vi "queryPanels (SubVI).vi"(4 "ThreatSize_0":refnum<vi>, 6 "Requestors_0":refnum<vi>, 7 "append":bool, 8 "error in":errorcluster, 9 "srchParams":T2={"maxPanels"=1001, "lkupPanelStartDate"=timestamp(0 s since 1904-01-01), "lkupPanelEndDate"=timestamp(0 s since 1904-01-01)} caption="Search Params" {"lkupPanelEndDate" format="%<%x>T"; "lkupPanelStartDate" format="%<%x>T"; "maxPanels" min=1 max=10000 step=100}, 10 "recoSet_IN":string[][](array[string]), 11 "criteria":T1) -> (0 "error out":errorcluster, 2 "recoSet_OUT":string[][](array[string]), 3 "actualNumPanels":i32)   [LabVIEW 2015]
panel:
  out "queryStr":string
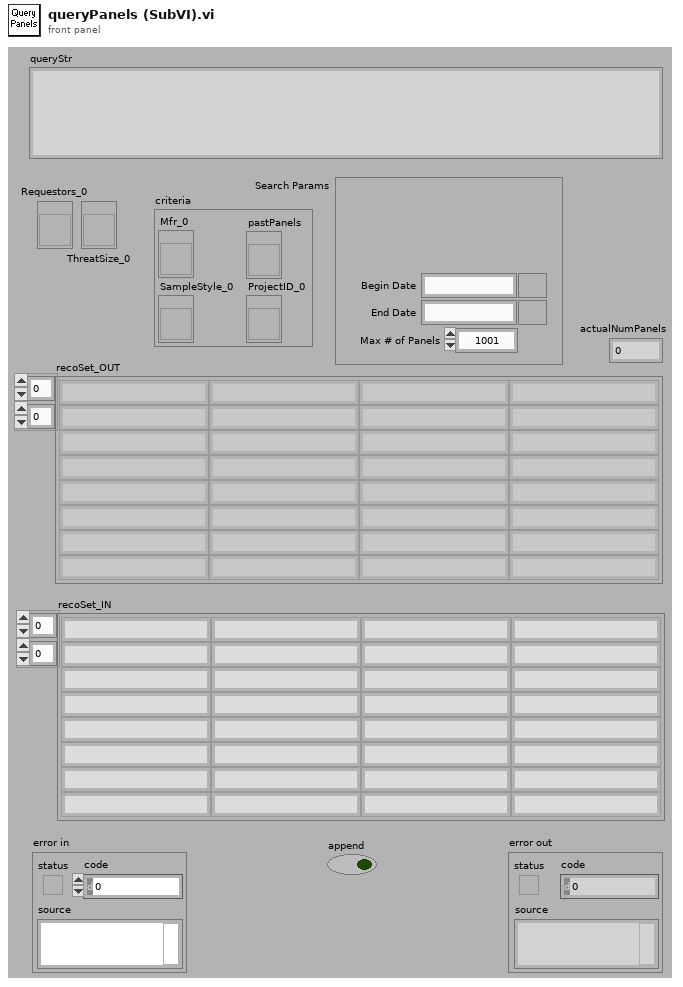
[diagram p1: front panel]
types:
  T1 = cluster{"Mfr_0":refnum<vi>, "SampleStyle_0":refnum<vi>, "pastPanels":refnum<vi>, "ProjectID_0":refnum<vi>}
  T2 = cluster{"maxPanels":u16, "lkupPanelStartDate":timestamp, "lkupPanelEndDate":timestamp}
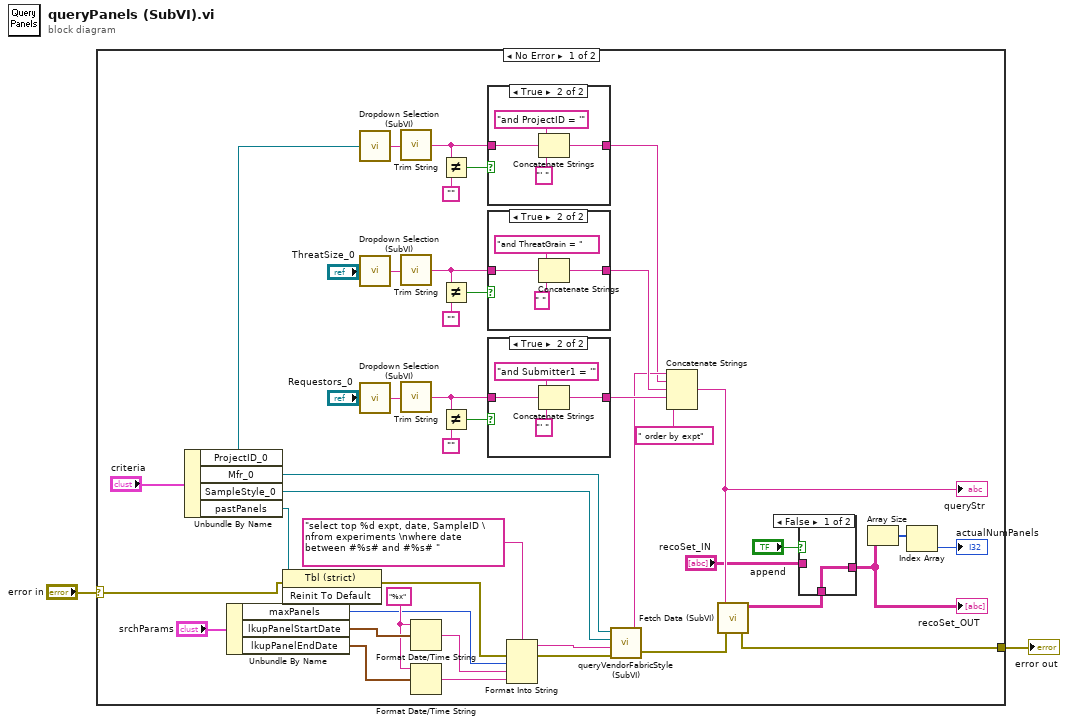
[diagram p0: block diagram]
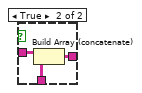
[diagram p2: hidden frame]
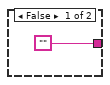
[diagram p3: hidden frame]
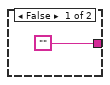
[diagram p4: hidden frame]
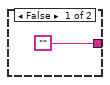
[diagram p5: hidden frame]
diagram:
  n1 = case shown="No Error" "error in" {
    selector: "error in" -> [w31 w67]
    tunnel: [w42 w67] -> w2
    frame No Error {
      w44 = "%x" ("time format string (%c)")
      n2 = Unbundle By Name("criteria") -> ("ProjectID_0"=w3:refnum<vi>, "Mfr_0"=w6:refnum<vi>, "SampleStyle_0"=w5:refnum<vi>, "pastPanels"=w4:refnum<vi>)
      n3 = Unbundle By Name("srchParams") -> ("maxPanels"=w38:u16, "lkupPanelStartDate"=w46:timestamp, "lkupPanelEndDate"=w47:timestamp)
      n4 = invoke class="Tbl (strict)" method="Reinit To Default"(reference=w4, error in=w31) -> (error out=w37:errorcluster)  [unwired: 1 in, 2 out]
      n5 = call "Dropdown Selection (SubVI).vi"("reference"=w3) -> ("element"=w17:string)
      n6 = call "Dropdown Selection (SubVI).vi"("reference"="ThreatSize_0") -> ("element"=w20:string)
      n7 = call "Dropdown Selection (SubVI).vi"("reference"="Requestors_0") -> ("element"=w29:string)
      n8 = call "Trim String.vi"("inStr"=w17) -> ("outStr"=w15:string)
      n9 = call "Trim String.vi"("inStr"=w20) -> ("outStr"=w22:string)
      n10 = call "Trim String.vi"("inStr"=w29) -> ("outStr"=w26:string)
      n11 = Format Date/Time String(time format string (%c)=w44, seconds (now)=w46) -> (date/time string=w39:string)  [unwired: 1 out]
      n12 = Format Date/Time String(time format string (%c)=w44, seconds (now)=w47) -> (date/time string=w40:string)  [unwired: 1 out]
      n13 = Not Equal?(x=w15, y="") -> (x != y?=w14:bool)
      n14 = Not Equal?(x=w22, y="") -> (x != y?=w23:bool)
      n15 = Not Equal?(x=w26, y="") -> (x != y?=w24:bool)
      n16 = case shown="True" w14 {
        tunnel: w15 -> [_ w54]
        tunnel: ["" w53] -> w12
        frame False {
        }
        frame True {
          n17 = Concatenate Strings("and ProjectID = '" ("Format String"), w54, "' " ("Format String")) -> (w53:string)
        }
      }
      n18 = case shown="True" w23 {
        tunnel: w22 -> [_ w59]
        tunnel: ["" w58] -> w18
        frame False {
        }
        frame True {
          n19 = Concatenate Strings("and ThreatGrain = " ("Format String"), w59, " " ("Format String")) -> (w58:string)
        }
      }
      n20 = case shown="True" w24 {
        tunnel: w26 -> [_ w64]
        tunnel: ["" w63] -> w25
        frame False {
        }
        frame True {
          n21 = Concatenate Strings("and Submitter1 = '" ("Format String"), w64, "' " ("Format String")) -> (w63:string)
        }
      }
      n22 = Format Into String(format string="select top %d expt, date, SampleID \nfrom experiments \nwhere date between #%s# and #%s# " ("Format String"), error in=w37, w38, w39, w40) -> (resulting string=w32:string, error out=w33:errorcluster)  [unwired: 1 in]
      n23 = call "queryVendorFabricStyle (SubVI).vi"("errorIn"=w33, "queryInStr"=w32, "SampleStyle_0"=w5, "Mfr_0"=w6) -> ("errorOut"=w34:errorcluster, "queryOutStr"=w13:string)
      n24 = Concatenate Strings(w13, w12, w18, w25, " order by expt" ("Format String")) -> (w35:string)
      "queryStr" <- w35
      n25 = call "Fetch Data (SubVI).vi"("error IN"=w34, "query string"=w35) -> ("error OUT"=w42:errorcluster, "recordset data"=w11:string[][])  [unwired: 4 out]
      n26 = case shown="False" "append" {
        tunnel: w11 -> [w48 w51]
        tunnel: [w48 w50] -> w10
        tunnel: "recoSet_IN" -> [_ w49]
        frame False {
        }
        frame True {
          n27 = Build Array (concatenate)(w49, w51) -> (w50:string[][])
        }
      }
      "recoSet_OUT" <- w10
      n28 = Array Size(array=w10) -> (size(s)=w43:i32[])
      n29 = Index Array(array=w43) -> (element=→"actualNumPanels":i32)  [unwired: 1 in]
    }
    frame Error {
    }
  }
  "error out" <- w2
